vi "API - Have All Errors Been Read.vi"(8 "Error In":errorcluster) -> (0 "Error Out":errorcluster, 3 "Have All Errors Been Read?":bool)   [LabVIEW 2023, in "Error Manager.lvlib"]
doc: "Returns a boolean that indicates whether all errors have been marked as read by the user.\n\nThe Boolean is TRUE if all errors have been marked as read OR if no errors have yet been reported to the asynchronous module.\nThe Boolean is FALSE otherwise (if there is at least one unread error).\n\nError in behaviour: This VI executes even if 'error in' contains an error."
uses:
  Error Manager.lvlib
  All Errors Read (library variable).vi
panel:
  # "Input\nInputs to the VI"
  # "Development\nControls or indicators that are useful for development or testing, but which are not outputs of the VI."
  # "Output\nOutputs of the VI"
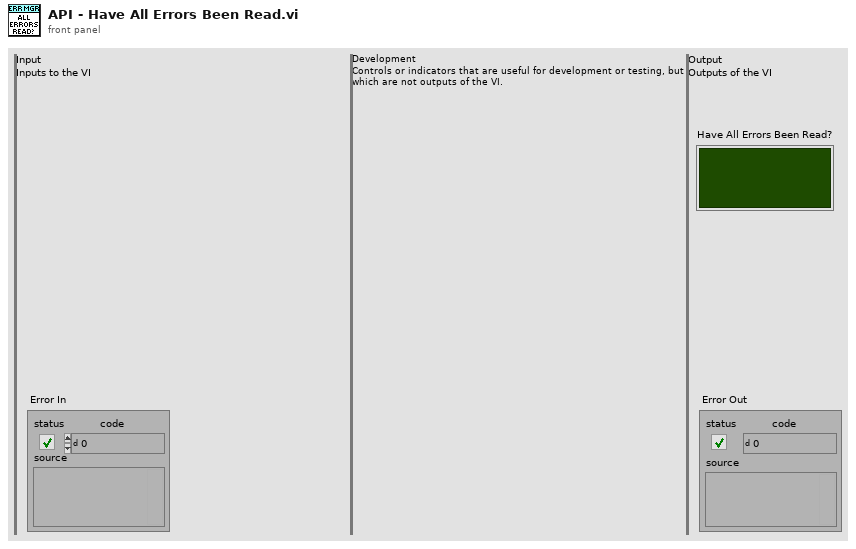
[diagram p1: front panel]
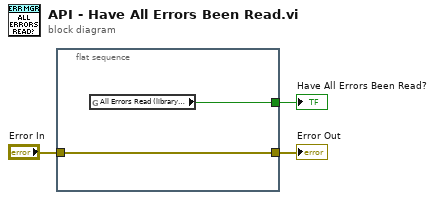
[diagram p0: block diagram]
diagram:
  n1 = flat-sequence {
    tunnel: [w5] -> w3
    tunnel: [w4] -> w2
    tunnel: "Error In" -> [w4]
    frame #0 {
      n2 = global read "All Errors Read (library variable).vi" item#0() -> (w5:bool)
    }
  }
  "Error Out" <- w2
  "Have All Errors Been Read?" <- w3
